vi "get power settings.vi"(8 "error in (no error)":errorcluster, 10 "power_settings":T1, 11 "id":i32) -> (0 "error out":errorcluster, 2 "power_settings out":T1, 3 "function return":i32)   [LabVIEW 2012, in "libximc.lvlib"]
doc: "result_t XIMC_API get_power_settings (device_t id, power_settings_t* power_settings);"
uses:
  libximc.lvlib
  libximc.dll
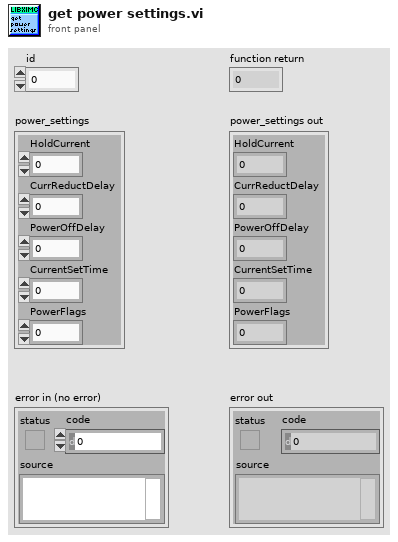
[diagram p1: front panel]
types:
  T1 = cluster{"HoldCurrent":u32, "CurrReductDelay":u32, "PowerOffDelay":u32, "CurrentSetTime":u32, "PowerFlags":u32}
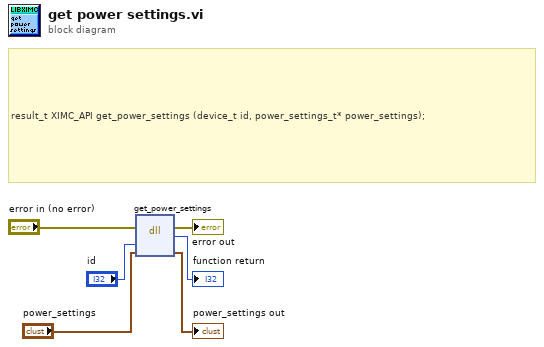
[diagram p0: block diagram]
diagram:
  # "result_t XIMC_API get_power_settings (device_t id, power_settings_t* power_settings);"
  n1 = dll-call lib="C:/Users/Vasily/Att_examples/LabVIEW_example/libximc.*" fn="get_power_settings"(error in="error in (no error)", "id"="id", "power_settings"="power_settings") -> (error out=→"error out":errorcluster, →"function return":i32, "power_settings"=→"power_settings out":T1)  [unwired: 3 in, 1 out]
